vi "Configure Digitizer Trigger.vi"(8 "error in (no error)":errorcluster, 9 "Post Trigger (0 %)":i32, 10 "Trigger Source (0: Auto)":i32(ring) items=["Auto", "RcvAC1", "RcvBC1", "RcvBlkC1", "RcvErrC1", "RcvAC2", "RcvBC2", "RcvBlkC2", "RcvErrC2", "RcvARef", "RcvBRef", "RcvBlkRef", "RcvErrRef", "XmtA", "XmtB", "XmitBlk", "RefOutA", "RefOutB", "RefOutBlk", "Generator", "ExtRise", "ExtFall"], 11 "VISA resource name":refnum<visa-resource-name>) -> (0 "error out":errorcluster, 3 "VISA resource name out":refnum<visa-resource-name>)   [LabVIEW 2014, in "Stanford Research SR1.lvlib"]
doc: "Configures attributes of the Digitizer Trigger."
uses:
  Stanford Research SR1.lvlib
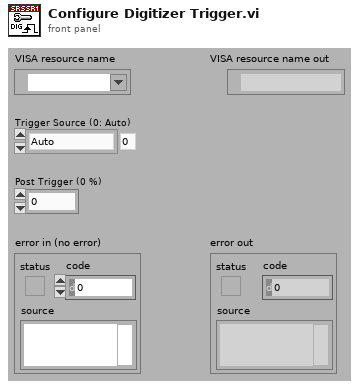
[diagram p1: front panel]
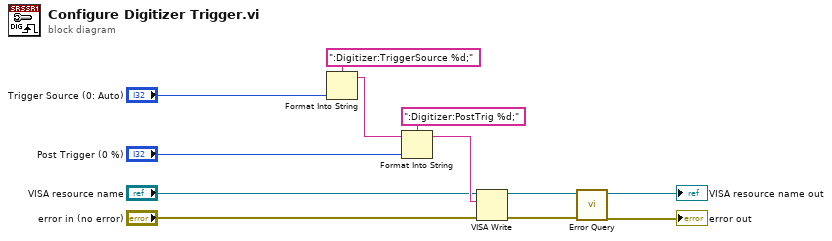
[diagram p0: block diagram]
diagram:
  n1 = Format Into String(format string=":Digitizer:TriggerSource %d;", "Trigger Source (0: Auto)") -> (resulting string=w10:string)  [unwired: 2 in, 1 out]
  n2 = Format Into String(format string=":Digitizer:PostTrig %d;", initial string=w10, "Post Trigger (0 %)") -> (resulting string=w7:string)  [unwired: 1 in, 1 out]
  n3 = VISA Write(VISA resource name="VISA resource name", write buffer=w7, error in (no error)="error in (no error)") -> (VISA resource name out=w4:refnum<visa-resource-name>, error out=w3:errorcluster)  [unwired: 1 out]
  n4 = call "Error Query.vi"("error in (no error)"=w3, "VISA resource name"=w4) -> ("error out"=→"error out":errorcluster, "VISA resource name out"=→"VISA resource name out":refnum<visa-resource-name>)  [unwired: 6 in, 2 out]
